vi "Clear Image.vi"(8 "error in":errorcluster, 11 "IMG_SRC in":refnum<class "IMG_SRC.lvclass">) -> (0 "error out":errorcluster, 3 "IMG_SRC out":refnum<class "IMG_SRC.lvclass">)   [LabVIEW 2018, in "IMG_SRC.lvlib" / "IMG_SRC.lvclass"]
uses:
  IMG_SRC.lvclass
  builds/Camera.lvlibp/Camera.lvclass
  C:/Users/Ron.Dexter.LUMINARTECH/Desktop/builds/Camera.lvlibp/Camera.lvclass
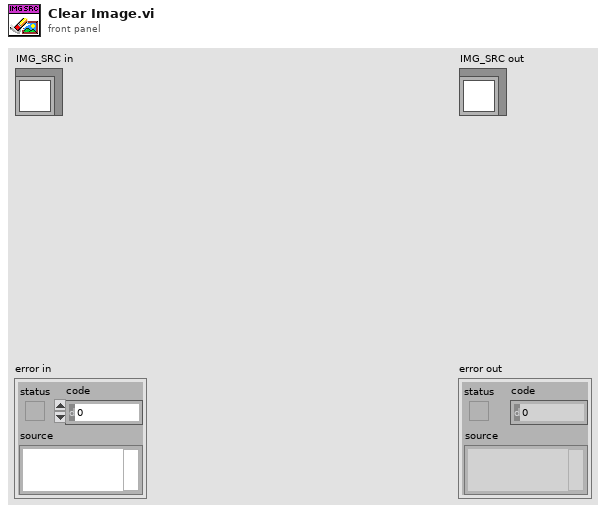
[diagram p1: front panel]
types:
  T1 = typedef "Camera.lvlibp/IMAQ Image.ctl" = refnum<image>
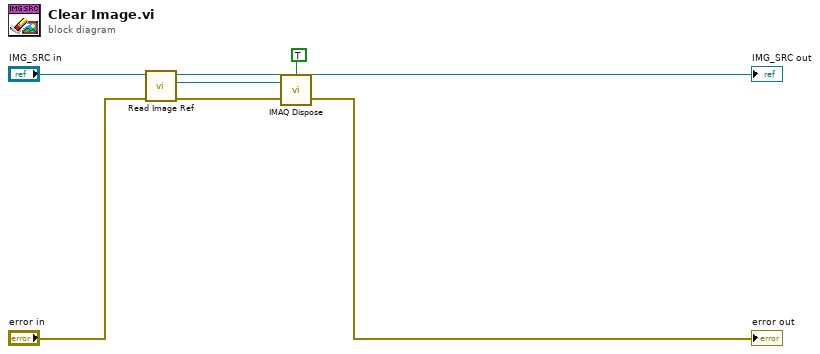
[diagram p0: block diagram]
diagram:
  n1 = call "Read Image Ref.vi"("error in (no error)"="error in", "Camera in"="IMG_SRC in") -> ("error out"=w2:errorcluster, "Image"=w1:T1, "Camera out"=→"IMG_SRC out":refnum<class "IMG_SRC.lvclass">)  [unwired: 7 in]
  n2 = call "IMAQ Dispose"("All Images? (No)"=TRUE, "Image"=w1, "error in (no error)"=w2) -> ("error out"=→"error out":errorcluster)  [unwired: 3 in]
